vi "Format Fast Data Files.vi"() -> ()   [LabVIEW 2013]
uses:
  <vilib>/Utility/file.llb/Read From Spreadsheet File (string).vi
panel:
  out "Correct":bool
  out "Calculated Freq (Hz)":i32
  in  "stop":bool
  in  "FileName":path caption="Fast Data File to Convert Time"
  out "~Percent Formatted":dbl
  out "Processing File":bool
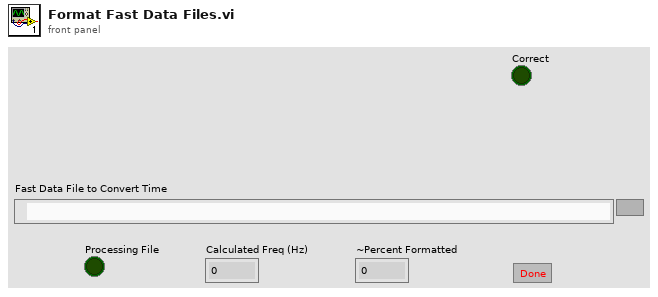
[diagram p1: front panel]
types:
  T1 = cluster{"Application":refnum<k7>, "Workbooks":refnum<k7>, "Workbook 1":refnum<k7>, "Sheets 1":refnum<k7>, "Worksheet 1":refnum<k7>, "Workbook 2":refnum<k7>, "Sheets 2":refnum<k7>, "Worksheet 2":refnum<k7>}
  T2 = cluster{"OrigFile":path, "NewFile":string, "AveFile":string, "RowIndex":i32, "Data":dbl[][], "Row#s/100":dbl, "Ave.ingLength":i32, "ExcelReferences":cluster{"Application":refnum<k7>, "Workbooks":refnum<k7>, "Workbook 1":refnum<k7>, "Sheets 1":refnum<k7>, "Worksheet 1":refnum<k7>, "Workbook 2":refnum<k7>, "Sheets 2":refnum<k7>, "Worksheet 2":refnum<k7>}, "Cells Hz":refnum<k7>, "Cells Ave":refnum<k7>, "Ave.ingPts":i32}
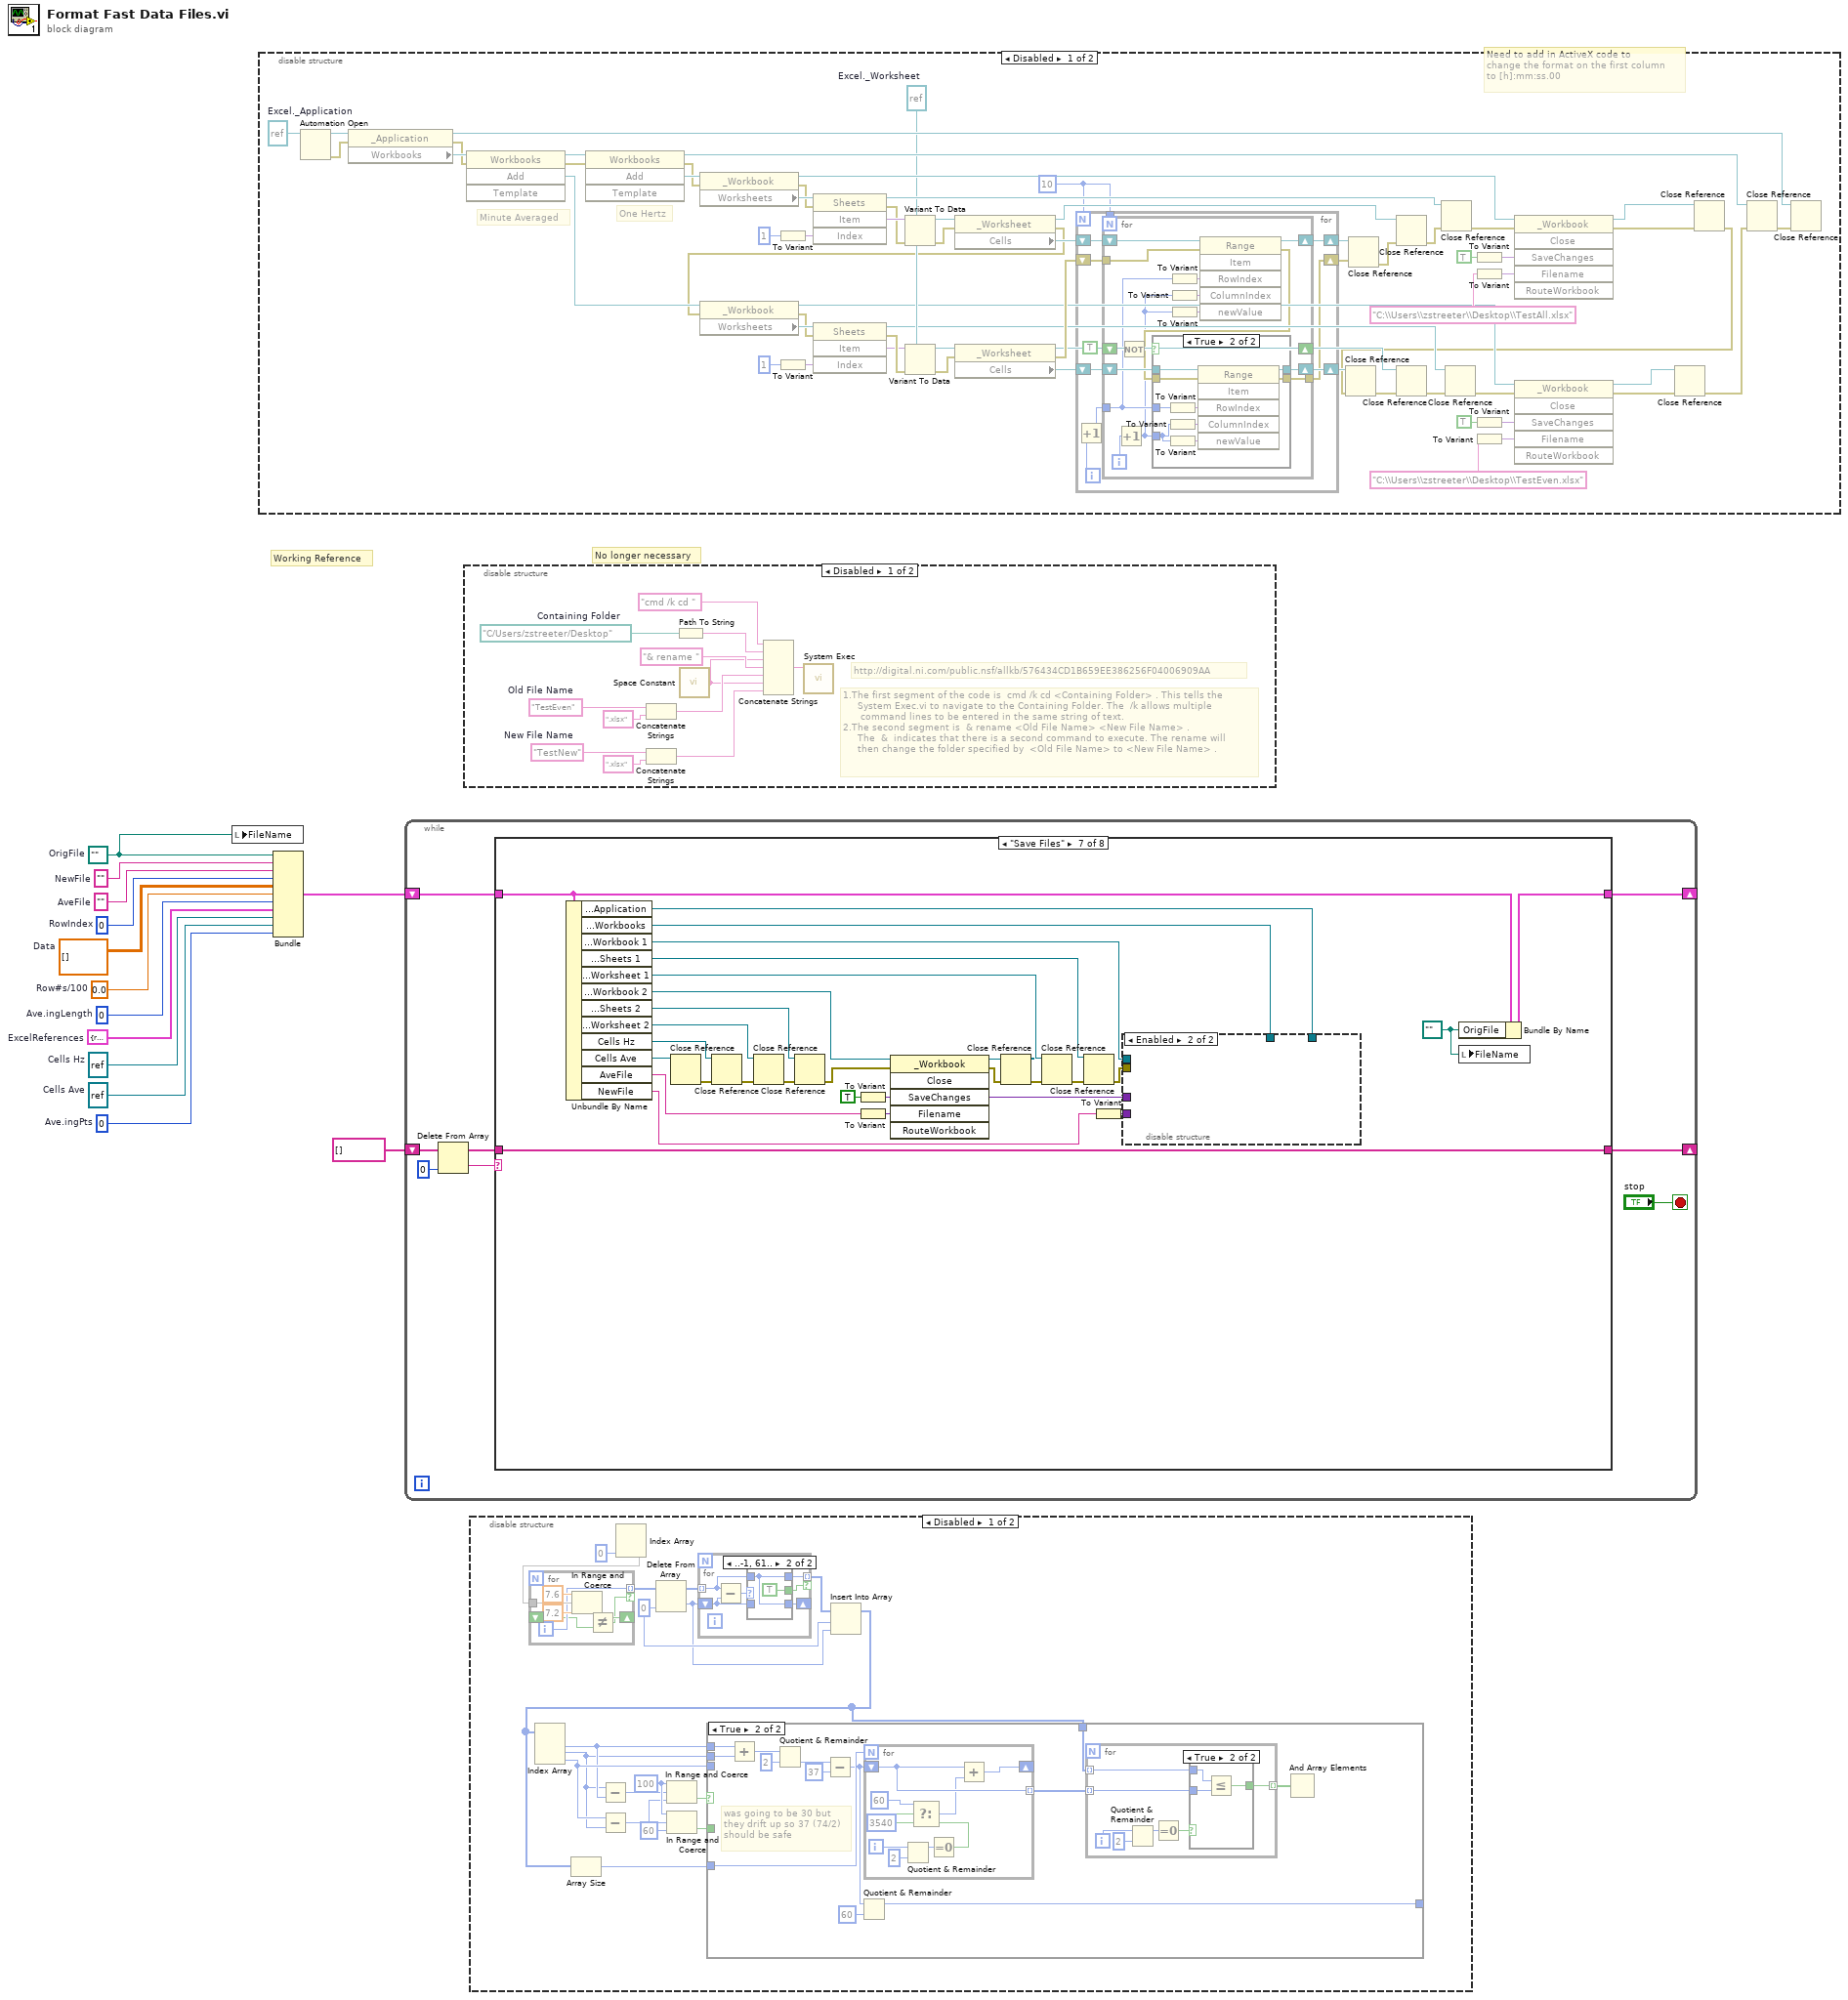
[diagram p0: block diagram]
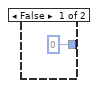
[diagram p2: hidden frame]
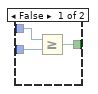
[diagram p3: hidden frame]
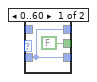
[diagram p4: hidden frame]
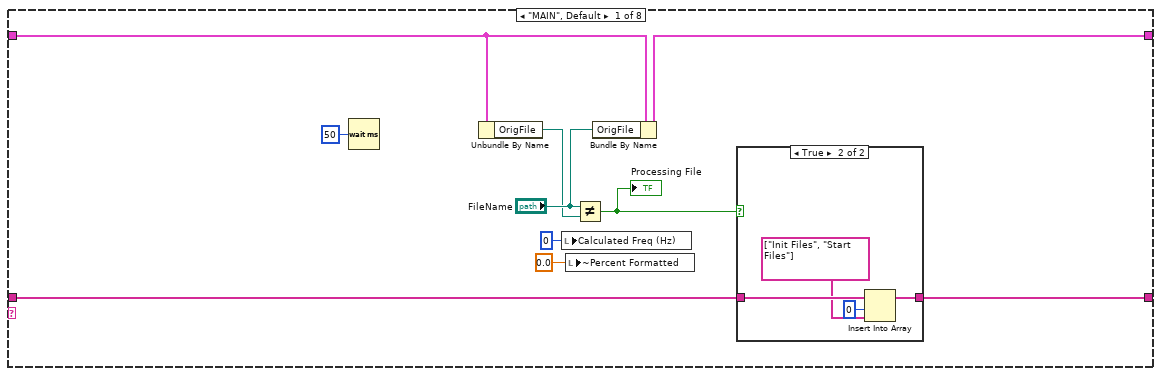
[diagram p6: hidden frame]
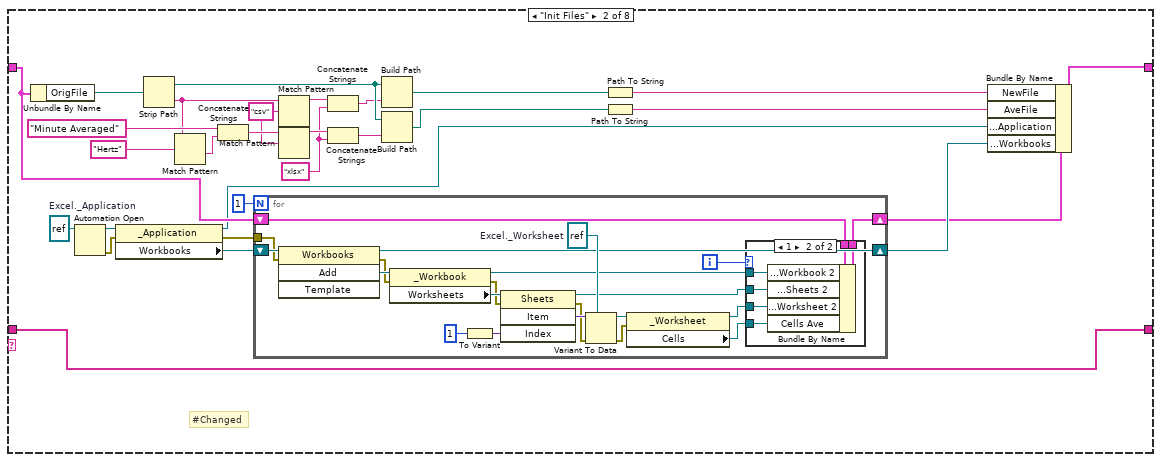
[diagram p8: hidden frame]
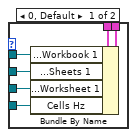
[diagram p9: hidden frame]
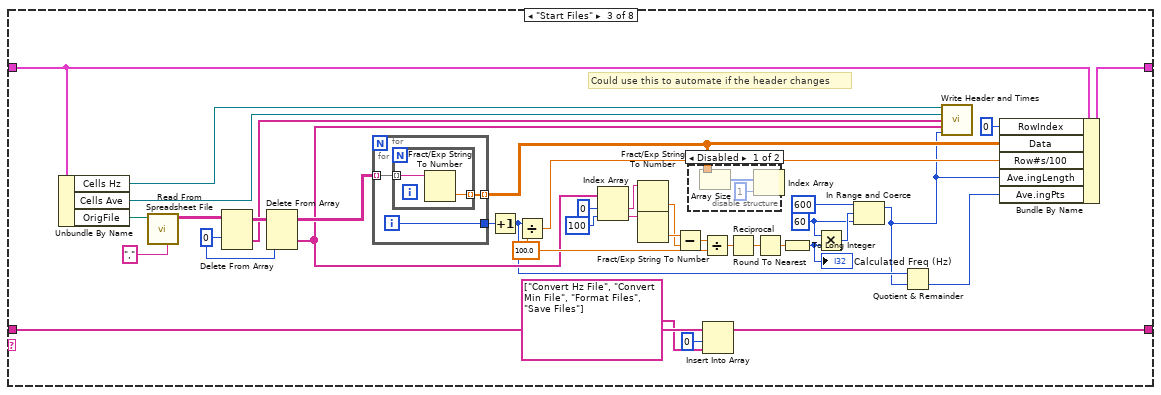
[diagram p10: hidden frame]
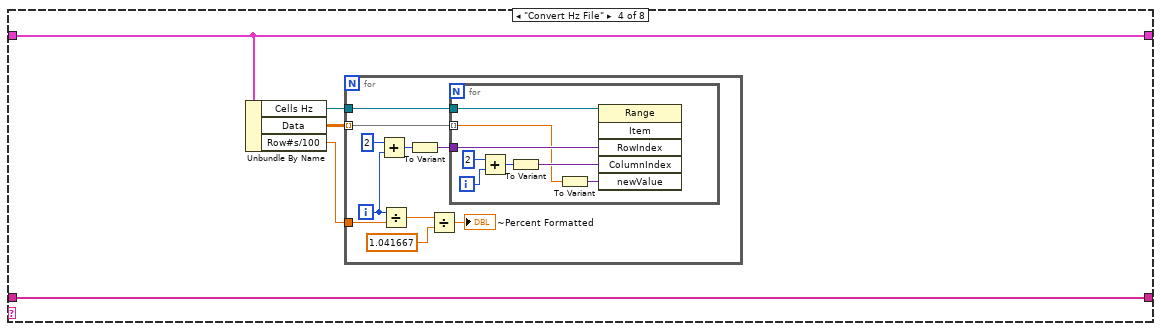
[diagram p12: hidden frame]
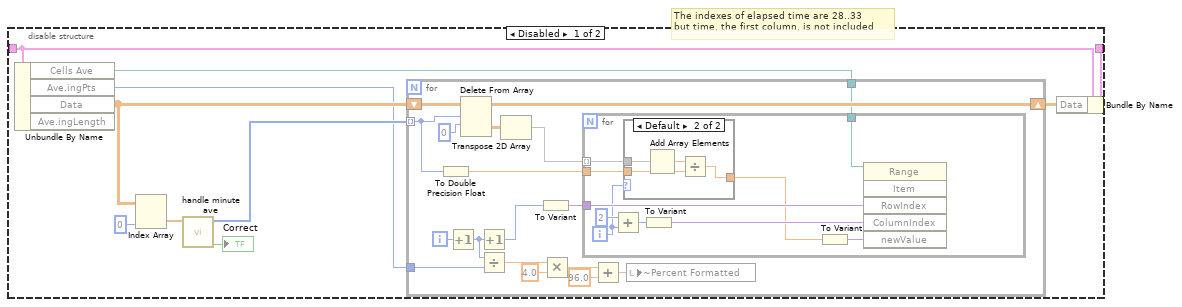
[diagram p14: hidden frame]
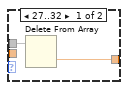
[diagram p15: hidden frame]
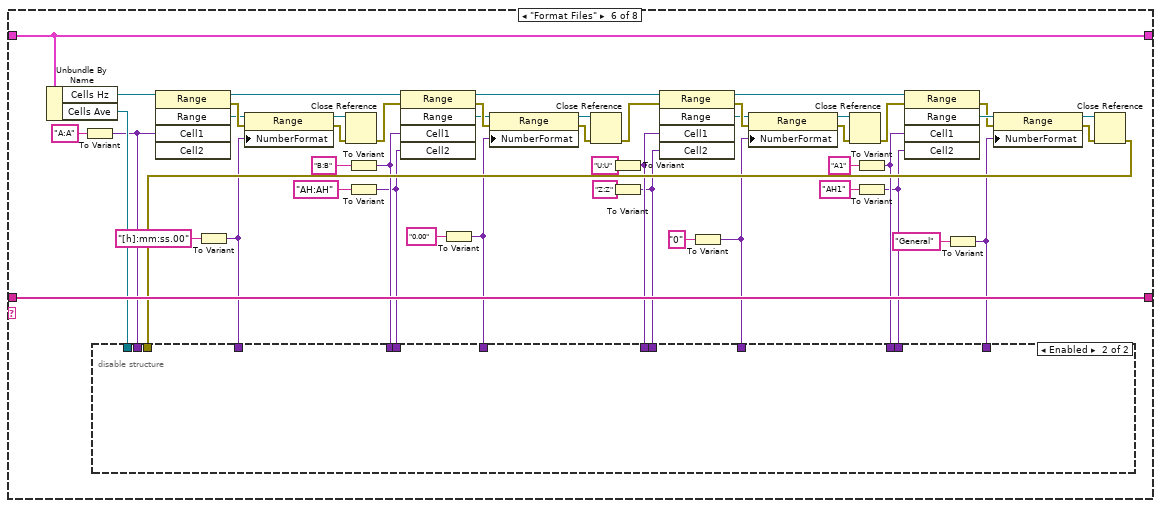
[diagram p16: hidden frame]
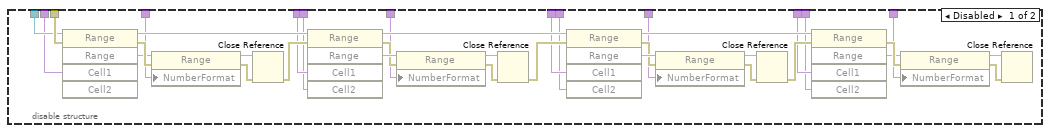
[diagram p17: hidden frame]
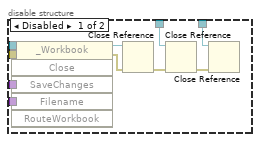
[diagram p18: hidden frame]
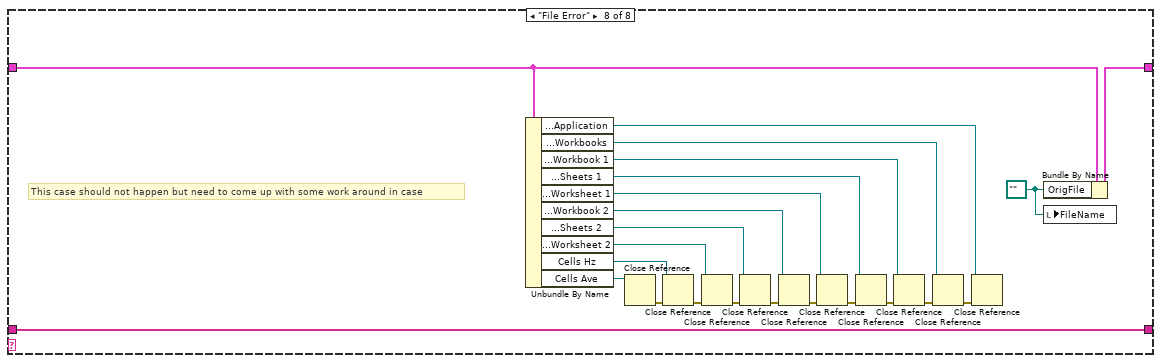
[diagram p19: hidden frame]
diagram:
  w3 = 0  # Ave.ingPts
  w5 = ""  # AveFile
  w4 = ""  # NewFile
  w6 = refnum<k7> refnum  # Cells Ave
  w7 = refnum<k7> refnum  # Cells Hz
  w8 = T1 {"Application"=refnum, "Workbooks"=refnum, "Workbook 1"=refnum, "Sheets 1"=refnum, "Worksheet 1"=refnum, "Workbook 2"=refnum, "Sheets 2"=refnum, "Worksheet 2"=refnum}  # ExcelReferences
  w10 = 0  # Ave.ingLength
  w9 = dbl[][] []  # Data
  w12 = 0  # RowIndex
  w11 = 0.0  # Row#s/100
  w2 = path ""  # OrigFile
  # "Working Reference"
  # "No longer necessary"
  n1 = local write "FileName"(w2) -> ()
  n2 = disable-structure shown="Disabled" {
    frame Disabled {
      w29 = 10
      w38 = refnum<k7> refnum  # Excel._Worksheet
      w77 = refnum<k7> refnum  # Excel._Application
      # "Need to add in ActiveX code to\nchange the format on the first column\nto [h]:mm:ss.00"
      # "Minute Averaged"
      # "One Hertz"
      n3 = Automation Open(Automation Refnum=w77) -> (Automation Refnum=w75:refnum<k7>, error out=w71:errorcluster)  [unwired: 3 in]
      n4 = property class="_Application"(reference=w75, error in=w71) -> (reference out=w64:refnum<k7>, error out=w48:errorcluster, "Workbooks"=w49:refnum<k7>)
      n5 = invoke class="Workbooks" method="Add"(reference=w49, error in=w48) -> (reference out=w46:refnum<k7>, error out=w47:errorcluster, "Add"=w45:refnum<k7>)  [unwired: 2 in, 1 out]
      n6 = invoke class="Workbooks" method="Add"(reference=w46, error in=w47) -> (reference out=w66:refnum<k7>, error out=w70:errorcluster, "Add"=w74:refnum<k7>)  [unwired: 2 in, 1 out]
      n7 = property class="_Workbook"(reference=w74, error in=w70) -> (reference out=w56:refnum<k7>, error out=w62:errorcluster, "Worksheets"=w63:refnum<k7>)
      n8 = To Variant(anything=1) -> (Variant=w59:variant)
      n9 = To Variant(anything=1) -> (Variant=w44:variant)
      n10 = invoke class="Sheets" method="Item"(reference=w63, error in=w62, "Index"=w59) -> (reference out=w67:refnum<k7>, error out=w69:errorcluster, "Item"=w72:variant)  [unwired: 1 in, 1 out]
      n11 = Variant To Data(error in=w69, type=w38, Variant=w72) -> (data=w61:refnum<k7>, error out=w68:errorcluster)
      n12 = property class="_Worksheet"(reference=w61, error in=w68) -> (reference out=w34:refnum<k7>, error out=w37:errorcluster, "Cells"=w60:refnum<k7>)
      n13 = property class="_Workbook"(reference=w45, error in=w37) -> (reference out=w19:refnum<k7>, error out=w41:errorcluster, "Worksheets"=w42:refnum<k7>)
      n14 = invoke class="Sheets" method="Item"(reference=w42, error in=w41, "Index"=w44) -> (reference out=w24:refnum<k7>, error out=w40:errorcluster, "Item"=w39:variant)  [unwired: 1 in, 1 out]
      n15 = Variant To Data(error in=w40, type=w38, Variant=w39) -> (data=w36:refnum<k7>, error out=w35:errorcluster)
      n16 = property class="_Worksheet"(reference=w36, error in=w35) -> (reference out=w25:refnum<k7>, error out=w31:errorcluster, "Cells"=w32:refnum<k7>)
      n17 = for {
        N: w29 -> [_]
        shift-right: [w86] -> w33
        shift-left: w60 -> [w87]
        shift-right: [w84] -> w28
        shift-left: w32 -> [w85]
        shift-right: [w81] -> w30
        shift-left: w31 -> [w82]
        tunnel: w29 -> [w78]
        i -> [w80]
        n18 = Increment(x=w80) -> (x+1=w79:i32)
        n19 = for {
          N: w78 -> [_]
          shift-right: [w98] -> w86
          shift-left: w87 -> [w102]
          shift-right: [w94] -> w84
          shift-left: w85 -> [w95]
          shift-right: [w96] -> _
          shift-left: TRUE -> [w97]
          tunnel: w82 -> [w93]
          tunnel: [w91] -> w81
          tunnel: w79 -> [w90]
          i -> [w89]
          n20 = Increment(x=w89) -> (x+1=w88:i32)
          n21 = Not(x=w97) -> (.not. x?=w96:bool)
          n22 = To Variant(anything=w90) -> (Variant=w99:variant)
          n23 = To Variant(anything=w88) -> (Variant=w100:variant)
          n24 = To Variant(anything=w88) -> (Variant=w101:variant)
          n25 = invoke class="Range" method="Item"(reference=w102, error in=w93, "RowIndex"=w99, "ColumnIndex"=w100, "newValue"=w101) -> (reference out=w98:refnum<k7>, error out=w92:errorcluster)  [unwired: 1 in, 4 out]
          n26 = case shown="True" w96 {
            tunnel: w95 -> [w104 w110]
            tunnel: [w104 w109] -> w94
            tunnel: w92 -> [w103 w108]
            tunnel: [w103 w107] -> w91
            tunnel: w90 -> [_ w106]
            tunnel: w88 -> [_ w105]
            frame False {
            }
            frame True {
              n27 = To Variant(anything=w106) -> (Variant=w113:variant)
              n28 = To Variant(anything=w105) -> (Variant=w112:variant)
              n29 = To Variant(anything=w105) -> (Variant=w111:variant)
              n30 = invoke class="Range" method="Item"(reference=w110, error in=w108, "RowIndex"=w113, "ColumnIndex"=w112, "newValue"=w111) -> (reference out=w109:refnum<k7>, error out=w107:errorcluster)  [unwired: 1 in, 4 out]
            }
          }
        }
      }
      n31 = Close Reference(reference=w33, error in (no error)=w30) -> (error out=w58:errorcluster)
      n32 = Close Reference(reference=w34, error in (no error)=w58) -> (error out=w76:errorcluster)
      n33 = Close Reference(reference=w67, error in (no error)=w76) -> (error out=w55:errorcluster)
      n34 = To Variant(anything=TRUE) -> (Variant=w51:variant)
      n35 = To Variant(anything="C:\\Users\\zstreeter\\Desktop\\TestAll.xlsx") -> (Variant=w52:variant)
      n36 = To Variant(anything=TRUE) -> (Variant=w22:variant)
      n37 = To Variant(anything="C:\\Users\\zstreeter\\Desktop\\TestEven.xlsx") -> (Variant=w21:variant)
      n38 = invoke class="_Workbook" method="Close"(reference=w56, error in=w55, "SaveChanges"=w51, "Filename"=w52) -> (reference out=w54:refnum<k7>, error out=w53:errorcluster)  [unwired: 2 in, 4 out]
      n39 = Close Reference(reference=w54, error in (no error)=w53) -> (error out=w15:errorcluster)
      n40 = Close Reference(reference=w28, error in (no error)=w15) -> (error out=w27:errorcluster)
      n41 = Close Reference(reference=w25, error in (no error)=w27) -> (error out=w26:errorcluster)
      n42 = Close Reference(reference=w24, error in (no error)=w26) -> (error out=w18:errorcluster)
      n43 = invoke class="_Workbook" method="Close"(reference=w19, error in=w18, "SaveChanges"=w22, "Filename"=w21) -> (reference out=w17:refnum<k7>, error out=w16:errorcluster)  [unwired: 2 in, 4 out]
      n44 = Close Reference(reference=w17, error in (no error)=w16) -> (error out=w14:errorcluster)
      n45 = Close Reference(reference=w66, error in (no error)=w14) -> (error out=w65:errorcluster)
      n46 = Close Reference(reference=w64, error in (no error)=w65) -> ()  [unwired: 1 out]
    }
    frame Enabled {
    }
  }
  n47 = Bundle("OrigFile"=w2, "NewFile"=w4, "AveFile"=w5, "RowIndex"=w12, "Data"=w9, "Row#s/100"=w11, "Ave.ingLength"=w10, "ExcelReferences"=w8, "Cells Hz"=w7, "Cells Ave"=w6, "Ave.ingPts"=w3) -> (w13:T2)  [unwired: 1 in]
  n48 = while {
    shift-right: [w117] -> _
    shift-left: string[] [] -> [w121]
    shift-right: [w115] -> _
    shift-left: w13 -> [w116]
    stop <- "stop" stop-if-true
    n49 = Delete From Array(array=w121, index=0) -> (deleted portion=w119:string, array with subset deleted=w118:string[])  [unwired: 1 in]
    n50 = case shown="\"Save Files\"" w119 {
      tunnel: w118 -> [w126 w164 w236 w249 w270 w364 w428 w461]
      tunnel: [w125 w164 w235 w249 w270 w364 w428 w461] -> w117
      tunnel: w116 -> [w130 w163 w234 w248 w269 w363 w427 w440]
      tunnel: [w129 w165 w233 w248 w268 w363 w426 w439] -> w115
      frame "MAIN", Default {
        n51 = Wait (ms)(milliseconds to wait=u32 50) -> ()  [unwired: 1 out]
        n52 = Unbundle By Name(w130) -> ("OrigFile"=w127:path)
        n53 = local write "Calculated Freq (Hz)"(0 ("Calculated Freq (Hz)")) -> ()
        n54 = local write "~Percent Formatted"(0.0 ("~Percent Formatted 2")) -> ()
        n55 = Not Equal?(x="FileName", y=w127) -> (x != y?=w124:bool)
        "Processing File" <- w124
        n56 = Bundle By Name(cluster=w130, "OrigFile"="FileName") -> (w129:T2)
        n57 = case shown="True" w124 {
          tunnel: w126 -> [w132 w136]
          tunnel: [w132 w135] -> w125
          frame False {
          }
          frame True {
            n58 = Insert Into Array(array=w136, index=0, new element=string[] ["Init Files", "Start Files"]) -> (w135:string[])
          }
        }
      }
      frame "Init Files" {
        w141 = refnum<k7> refnum  # Excel._Application
        w152 = "xlsx" ("regular expression")
        w156 = "csv" ("regular expression")
        # "#Changed"
        n59 = Unbundle By Name(w163) -> ("OrigFile"=w158:path)
        n60 = Automation Open(Automation Refnum=w141) -> (Automation Refnum=w142:refnum<k7>, error out=w143:errorcluster)  [unwired: 3 in]
        n61 = property class="_Application"(reference=w142, error in=w143) -> (reference out=w139:refnum<k7>, error out=w145:errorcluster, "Workbooks"=w144:refnum<k7>)
        n62 = Strip Path(path=w158) -> (stripped path=w162:path, name=w155:string)
        n63 = Match Pattern(string=w155, regular expression="Hertz") -> (after substring=w160:string)  [unwired: 1 in, 3 out]
        n64 = Concatenate Strings("Minute Averaged" ("string"), w160) -> (w157:string)
        n65 = for {
          N: 1 -> [_]
          shift-right: [w173] -> w140
          shift-left: w144 -> [w176]
          tunnel: w145 -> [w175]
          shift-right: [w171] -> w138
          shift-left: w163 -> [w172]
          i -> [w166]
          w174 = refnum<k7> refnum  # Excel._Worksheet
          n66 = invoke class="Workbooks" method="Add"(reference=w176, error in=w175) -> (reference out=w173:refnum<k7>, error out=w183:errorcluster, "Add"=w186:refnum<k7>)  [unwired: 2 in, 1 out]
          n67 = property class="_Workbook"(reference=w186, error in=w183) -> (reference out=w170:refnum<k7>, error out=w179:errorcluster, "Worksheets"=w180:refnum<k7>)
          n68 = To Variant(anything=1) -> (Variant=w177:variant)
          n69 = invoke class="Sheets" method="Item"(reference=w180, error in=w179, "Index"=w177) -> (reference out=w169:refnum<k7>, error out=w182:errorcluster, "Item"=w184:variant)  [unwired: 1 in, 1 out]
          n70 = Variant To Data(error in=w182, type=w174, Variant=w184) -> (data=w178:refnum<k7>, error out=w181:errorcluster)
          n71 = property class="_Worksheet"(reference=w178, error in=w181) -> (reference out=w168:refnum<k7>, "Cells"=w167:refnum<k7>)  [unwired: 1 out]
          n72 = case shown="1" w166 {
            tunnel: w172 -> [w192 w198]
            tunnel: [w191 w197] -> w171
            tunnel: w170 -> [w190 w196]
            tunnel: w169 -> [w189 w195]
            tunnel: w168 -> [w188 w194]
            tunnel: w167 -> [w187 w193]
            frame 0, Default {
              n73 = Bundle By Name(cluster=w192, "ExcelReferences.Workbook 1"=w190, "ExcelReferences.Sheets 1"=w189, "ExcelReferences.Worksheet 1"=w188, "Cells Hz"=w187) -> (w191:T2)
            }
            frame 1 {
              n74 = Bundle By Name(cluster=w198, "ExcelReferences.Workbook 2"=w196, "ExcelReferences.Sheets 2"=w195, "ExcelReferences.Worksheet 2"=w194, "Cells Ave"=w193) -> (w197:T2)
            }
          }
        }
        n75 = Match Pattern(string=w155, regular expression=w156) -> (before substring=w153:string)  [unwired: 1 in, 3 out]
        n76 = Match Pattern(string=w157, regular expression=w156) -> (before substring=w154:string)  [unwired: 1 in, 3 out]
        n77 = Concatenate Strings(w153, w152) -> (w150:string)
        n78 = Concatenate Strings(w154, w152) -> (w151:string)
        n79 = Build Path(base path=w162, name or relative path=w150) -> (appended path=w148:path)
        n80 = Build Path(base path=w162, name or relative path=w151) -> (appended path=w149:path)
        n81 = Path To String(path=w148) -> (string=w146:string)
        n82 = Path To String(path=w149) -> (string=w147:string)
        n83 = Bundle By Name(cluster=w138, "NewFile"=w146, "AveFile"=w147, "ExcelReferences.Application"=w139, "ExcelReferences.Workbooks"=w140) -> (w165:T2)
      }
      frame "Start Files" {
        w209 = 60 ("x")
        w204 = 100.0 ("y")
        w221 = 0 ("index (row)")
        # "Could use this to automate if the header changes"
        n84 = Unbundle By Name(w234) -> ("Cells Hz"=w228:refnum<k7>, "Cells Ave"=w229:refnum<k7>, "OrigFile"=w230:path)
        n85 = call-poly <vilib>:"Read From Spreadsheet File.vi"("delimiter (\\t)"="," ("delimiter (\\t)"), "file path (dialog if empty)"=w230) -> ("all rows"=w231:string[][])  [unwired: 5 in, 4 out]
        n86 = Delete From Array(array=w231, index (row)=w221) -> (deleted portion=w202:string[], array with subset deleted=w226:string[][])  [unwired: 2 in]
        n87 = Delete From Array(array=w226, index (col)=w221) -> (deleted portion=w203:string[], array with subset deleted=w222:string[][])  [unwired: 2 in]
        n88 = for {
          tunnel: w222 -> [w242] mode=indexing
          tunnel: [w241] -> w207 mode=indexing
          tunnel: [w240] -> w225
          i -> [w240]
          n89 = for {
            tunnel: w242 -> [w244] mode=indexing
            tunnel: [w243] -> w241 mode=indexing
            n90 = Fract/Exp String To Number(string=w244) -> (number=w243:dbl)  [unwired: 3 in, 1 out]
          }
        }
        n91 = Increment(x=w225) -> (x+1=w201:i32)
        n92 = Divide(x=w201, y=w204) -> (x/y=w205:dbl)
        n93 = Index Array(array=w203, index #1=0 ("index"), index #2=100 ("index")) -> (element #1=w218:string, element #2=w217:string)
        n94 = Fract/Exp String To Number(string=w218) -> (number=w215:dbl)  [unwired: 3 in, 1 out]
        n95 = Fract/Exp String To Number(string=w217) -> (number=w216:dbl)  [unwired: 3 in, 1 out]
        n96 = Subtract(x=w216, y=w215) -> (x-y=w214:dbl)
        n97 = disable-structure shown="Disabled" {
          disable-tunnel: w207 -> [w237 _]
          frame Disabled {
            n98 = Array Size(array=w237) -> (size(s)=w239:i32[])
            n99 = Index Array(array=w239, index=1) -> ()  [unwired: 1 out]
          }
          frame Enabled {
          }
        }
        n100 = Divide(x=w214, y=w204) -> (x/y=w213:dbl)
        n101 = Insert Into Array(array=w236, index=0, new element=string[] ["Convert Hz File", "Convert Min File", "Format Files", "Save Files"]) -> (w235:string[])
        n102 = Reciprocal(x=w213) -> (1/x=w212:dbl)
        n103 = Round To Nearest(number=w212) -> (nearest integer value=w211:dbl)
        n104 = To Long Integer(number=w211) -> (32bit integer=w206:i32)
        "Calculated Freq (Hz)" <- w206
        n105 = Multiply(x=w209, y=w206) -> (x*y=w210:i32)
        n106 = In Range and Coerce(upper limit=600, x=w210, lower limit=w209) -> (coerced(x)=w199:i32)  [unwired: 1 out]
        n107 = Quotient & Remainder(x=w201, y=w199) -> (floor(x/y)=w200:i32)  [unwired: 1 out]
        n108 = call "Write Header and Times.vi"("Cells Hz IN"=w228, "Cells Ave IN"=w229, "Header Array"=w202, "Time Array"=w203, "Ave.ingLength"=w199) -> ()  [unwired: 9 in, 2 out]
        n109 = Bundle By Name(cluster=w234, "RowIndex"=0, "Data"=w207, "Row#s/100"=w205, "Ave.ingLength"=w199, "Ave.ingPts"=w200) -> (w233:T2)
      }
      frame "Convert Hz File" {
        n110 = Unbundle By Name(w248) -> ("Cells Hz"=w245:refnum<k7>, "Data"=w247:dbl[][], "Row#s/100"=w246:dbl)
        n111 = for {
          tunnel: w247 -> [w259] mode=indexing
          tunnel: w246 -> [w255]
          tunnel: w245 -> [w252]
          i -> [w254]
          n112 = Add(x=2, y=w254) -> (x+y=w251:i32)
          n113 = Divide(x=w254, y=w255) -> (x/y=w256:dbl)
          n114 = To Variant(anything=w251) -> (Variant=w250:variant)
          n115 = Divide(x=w256, y=1.041667) -> (x/y=→"~Percent Formatted":dbl)
          n116 = for {
            tunnel: w259 -> [w260] mode=indexing
            tunnel: w252 -> [w267]
            tunnel: w250 -> [w266]
            i -> [w262]
            n117 = Add(x=2, y=w262) -> (x+y=w265:i32)
            n118 = To Variant(anything=w265) -> (Variant=w263:variant)
            n119 = To Variant(anything=w260) -> (Variant=w261:variant)
            n120 = invoke class="Range" method="Item"(reference=w267, "RowIndex"=w266, "ColumnIndex"=w263, "newValue"=w261) -> ()  [unwired: 2 in, 6 out]
          }
        }
      }
      frame "Convert Min File" {
        n121 = disable-structure shown="Enabled" {
          disable-tunnel: w269 -> [w280 w315]
          disable-tunnel: [w279 w315] -> w268
          frame Disabled {
            # "The indexes of elapsed time are 28..33\nbut time, the first column, is not included"
            n122 = Unbundle By Name(w280) -> ("Cells Ave"=w278:refnum<k7>, "Ave.ingPts"=w271:i32, "Data"=w275:dbl[][])  [unwired: 1 out]
            n123 = Index Array(array=w275, index (col)=0 ("disabled index (col)")) -> (element=w274:dbl[])  [unwired: 1 in]
            n124 = call "handle minute ave.vi"("Array"=w274) -> ("Correct"=→"Correct":bool, "Array 2"=w272:i32[])  [unwired: 9 in]
            n125 = for {
              shift-right: [w296] -> w277
              shift-left: w275 -> [w298]
              tunnel: w272 -> [w283] mode=indexing
              tunnel: w278 -> [w286]
              tunnel: w271 -> [w281]
              i -> [w295]
              n126 = To Double Precision Float(number=w283) -> (double precision float=w282:dbl)
              n127 = Increment(x=w295) -> (x+1=w294:i32)
              n128 = Delete From Array(array=w298, length=w283, index (row)=0) -> (deleted portion=w284:dbl[][], array with subset deleted=w296:dbl[][])  [unwired: 1 in]
              n129 = Increment(x=w294) -> (x+1=w289:i32)
              n130 = Divide(x=w294, y=w281) -> (x/y=w293:dbl)
              n131 = Transpose 2D Array(2D array=w284) -> (transposed array=w285:dbl[][])
              n132 = To Variant(anything=w289) -> (Variant=w290:variant)
              n133 = Multiply(x=w293, y=4.0) -> (x*y=w288:dbl)
              n134 = for {
                tunnel: w290 -> [w308]
                tunnel: w286 -> [w304]
                tunnel: w285 -> [w303] mode=indexing
                tunnel: w282 -> [w302]
                i -> [w301]
                n135 = Add(x=2, y=w301) -> (x+y=w307:i32)
                n136 = case shown="Default" w301 {
                  tunnel: w303 -> [w310 w313]
                  tunnel: w302 -> [_ w312]
                  tunnel: [w309 w311] -> w300
                  frame 27..32 {
                    n137 = Delete From Array(array=w310) -> (deleted portion=w309:dbl)  [unwired: 2 in, 1 out]
                  }
                  frame Default {
                    n138 = Add Array Elements(numeric array=w313) -> (sum=w314:dbl)
                    n139 = Divide(x=w314, y=w312) -> (x/y=w311:dbl)
                  }
                }
                n140 = To Variant(anything=w307) -> (Variant=w305:variant)
                n141 = To Variant(anything=w300) -> (Variant=w299:variant)
                n142 = invoke class="Range" method="Item"(reference=w304, "RowIndex"=w308, "ColumnIndex"=w305, "newValue"=w299) -> ()  [unwired: 2 in, 6 out]
              }
              n143 = Add(x=w288, y=96.0 ("x")) -> (x+y=w291:dbl)
              n144 = local write "~Percent Formatted"(w291) -> ()
            }
            n145 = Bundle By Name(cluster=w280, "Data"=w277) -> (w279:T2)
          }
          frame Enabled {
          }
        }
      }
      frame "Format Files" {
        n146 = Unbundle By Name(w363) -> ("Cells Hz"=w318:refnum<k7>, "Cells Ave"=w343:refnum<k7>)
        n147 = To Variant(anything="A:A") -> (Variant=w339:variant)
        n148 = invoke class="Range" method="Range"(reference=w318, "Cell1"=w339) -> (reference out=w317:refnum<k7>, error out=w362:errorcluster, "Range"=w316:refnum<k7>)  [unwired: 3 in, 2 out]
        n149 = To Variant(anything="[h]:mm:ss.00") -> (Variant=w325:variant)
        n150 = property class="Range"(reference=w316, error in=w362, "NumberFormat"=w325) -> (reference out=w360:refnum<k7>, error out=w361:errorcluster)
        n151 = Close Reference(reference=w360, error in (no error)=w361) -> (error out=w347:errorcluster)
        n152 = To Variant(anything="B:B") -> (Variant=w336:variant)
        n153 = To Variant(anything="AH:AH") -> (Variant=w335:variant)
        n154 = invoke class="Range" method="Range"(reference=w317, error in=w347, "Cell1"=w336, "Cell2"=w335) -> (reference out=w342:refnum<k7>, error out=w357:errorcluster, "Range"=w356:refnum<k7>)  [unwired: 1 in, 2 out]
        n155 = To Variant(anything="0.00") -> (Variant=w319:variant)
        n156 = property class="Range"(reference=w356, error in=w357, "NumberFormat"=w319) -> (reference out=w359:refnum<k7>, error out=w358:errorcluster)
        n157 = Close Reference(reference=w359, error in (no error)=w358) -> (error out=w346:errorcluster)
        n158 = To Variant(anything="U:U") -> (Variant=w328:variant)
        n159 = To Variant(anything="Z:Z") -> (Variant=w327:variant)
        n160 = invoke class="Range" method="Range"(reference=w342, error in=w346, "Cell1"=w328, "Cell2"=w327) -> (reference out=w341:refnum<k7>, error out=w349:errorcluster, "Range"=w348:refnum<k7>)  [unwired: 1 in, 2 out]
        n161 = To Variant(anything="0") -> (Variant=w320:variant)
        n162 = property class="Range"(reference=w348, error in=w349, "NumberFormat"=w320) -> (reference out=w351:refnum<k7>, error out=w350:errorcluster)
        n163 = Close Reference(reference=w351, error in (no error)=w350) -> (error out=w345:errorcluster)
        n164 = To Variant(anything="A1") -> (Variant=w330:variant)
        n165 = To Variant(anything="AH1") -> (Variant=w329:variant)
        n166 = invoke class="Range" method="Range"(reference=w341, error in=w345, "Cell1"=w330, "Cell2"=w329) -> (error out=w354:errorcluster, "Range"=w355:refnum<k7>)  [unwired: 1 in, 3 out]
        n167 = To Variant(anything="General") -> (Variant=w323:variant)
        n168 = property class="Range"(reference=w355, error in=w354, "NumberFormat"=w323) -> (reference out=w352:refnum<k7>, error out=w353:errorcluster)
        n169 = Close Reference(reference=w352, error in (no error)=w353) -> (error out=w344:errorcluster)
        n170 = disable-structure shown="Enabled" {
          disable-tunnel: w344 -> [w383 _]
          disable-tunnel: w343 -> [w379 _]
          disable-tunnel: w339 -> [w375 _]
          disable-tunnel: w336 -> [w374 _]
          disable-tunnel: w335 -> [w373 _]
          disable-tunnel: w330 -> [w372 _]
          disable-tunnel: w329 -> [w371 _]
          disable-tunnel: w328 -> [w370 _]
          disable-tunnel: w327 -> [w369 _]
          disable-tunnel: w325 -> [w368 _]
          disable-tunnel: w323 -> [w367 _]
          disable-tunnel: w320 -> [w366 _]
          disable-tunnel: w319 -> [w365 _]
          frame Disabled {
            n171 = invoke class="Range" method="Range"(reference=w379, error in=w383, "Cell1"=w375) -> (reference out=w378:refnum<k7>, error out=w385:errorcluster, "Range"=w384:refnum<k7>)  [unwired: 2 in, 2 out]
            n172 = property class="Range"(reference=w384, error in=w385, "NumberFormat"=w368) -> (reference out=w387:refnum<k7>, error out=w386:errorcluster)
            n173 = Close Reference(reference=w387, error in (no error)=w386) -> (error out=w382:errorcluster)
            n174 = invoke class="Range" method="Range"(reference=w378, error in=w382, "Cell1"=w374, "Cell2"=w373) -> (reference out=w377:refnum<k7>, error out=w390:errorcluster, "Range"=w391:refnum<k7>)  [unwired: 1 in, 2 out]
            n175 = property class="Range"(reference=w391, error in=w390, "NumberFormat"=w365) -> (reference out=w388:refnum<k7>, error out=w389:errorcluster)
            n176 = Close Reference(reference=w388, error in (no error)=w389) -> (error out=w381:errorcluster)
            n177 = invoke class="Range" method="Range"(reference=w377, error in=w381, "Cell1"=w370, "Cell2"=w369) -> (reference out=w376:refnum<k7>, error out=w398:errorcluster, "Range"=w399:refnum<k7>)  [unwired: 1 in, 2 out]
            n178 = property class="Range"(reference=w399, error in=w398, "NumberFormat"=w366) -> (reference out=w396:refnum<k7>, error out=w397:errorcluster)
            n179 = Close Reference(reference=w396, error in (no error)=w397) -> (error out=w380:errorcluster)
            n180 = invoke class="Range" method="Range"(reference=w376, error in=w380, "Cell1"=w372, "Cell2"=w371) -> (error out=w393:errorcluster, "Range"=w392:refnum<k7>)  [unwired: 1 in, 3 out]
            n181 = property class="Range"(reference=w392, error in=w393, "NumberFormat"=w367) -> (reference out=w395:refnum<k7>, error out=w394:errorcluster)
            n182 = Close Reference(reference=w395, error in (no error)=w394) -> ()  [unwired: 1 out]
          }
          frame Enabled {
          }
        }
      }
      frame "Save Files" {
        w400 = path "" ("OrigFile")
        n183 = Unbundle By Name(w427) -> ("ExcelReferences.Application"=w418:refnum<k7>, "ExcelReferences.Workbooks"=w419:refnum<k7>, "ExcelReferences.Workbook 1"=w409:refnum<k7>, "ExcelReferences.Sheets 1"=w420:refnum<k7>, "ExcelReferences.Worksheet 1"=w421:refnum<k7>, "ExcelReferences.Workbook 2"=w408:refnum<k7>, "ExcelReferences.Sheets 2"=w422:refnum<k7>, "ExcelReferences.Worksheet 2"=w423:refnum<k7>, "Cells Hz"=w424:refnum<k7>, "Cells Ave"=w425:refnum<k7>, "AveFile"=w402:string, "NewFile"=w401:string)
        n184 = Close Reference(reference=w425) -> (error out=w417:errorcluster)  [unwired: 1 in]
        n185 = Close Reference(reference=w424, error in (no error)=w417) -> (error out=w416:errorcluster)
        n186 = Close Reference(reference=w423, error in (no error)=w416) -> (error out=w415:errorcluster)
        n187 = Close Reference(reference=w422, error in (no error)=w415) -> (error out=w406:errorcluster)
        n188 = To Variant(anything=TRUE) -> (Variant=w403:variant)
        n189 = To Variant(anything=w402) -> (Variant=w411:variant)
        n190 = invoke class="_Workbook" method="Close"(reference=w408, error in=w406, "SaveChanges"=w403, "Filename"=w411) -> (reference out=w407:refnum<k7>, error out=w405:errorcluster)  [unwired: 2 in, 4 out]
        n191 = Close Reference(reference=w407, error in (no error)=w405) -> (error out=w414:errorcluster)
        n192 = Close Reference(reference=w421, error in (no error)=w414) -> (error out=w413:errorcluster)
        n193 = Close Reference(reference=w420, error in (no error)=w413) -> (error out=w404:errorcluster)
        n194 = To Variant(anything=w401) -> (Variant=w412:variant)
        n195 = disable-structure shown="Enabled" {
          disable-tunnel: w419 -> [w438 _]
          disable-tunnel: w418 -> [w437 _]
          disable-tunnel: w412 -> [w434 _]
          disable-tunnel: w409 -> [w433 _]
          disable-tunnel: w404 -> [w431 _]
          disable-tunnel: w403 -> [w429 _]
          frame Disabled {
            n196 = invoke class="_Workbook" method="Close"(reference=w433, error in=w431, "SaveChanges"=w429, "Filename"=w434) -> (reference out=w432:refnum<k7>, error out=w430:errorcluster)  [unwired: 2 in, 4 out]
            n197 = Close Reference(reference=w432, error in (no error)=w430) -> (error out=w436:errorcluster)
            n198 = Close Reference(reference=w438, error in (no error)=w436) -> (error out=w435:errorcluster)
            n199 = Close Reference(reference=w437, error in (no error)=w435) -> ()  [unwired: 1 out]
          }
          frame Enabled {
          }
        }
        n200 = Bundle By Name(cluster=w427, "OrigFile"=w400) -> (w426:T2)
        n201 = local write "FileName"(w400) -> ()
      }
      frame "File Error" {
        w441 = path "" ("OrigFile")
        # "This case should not happen but need to come up with some work around in case"
        n202 = Unbundle By Name(w440) -> ("ExcelReferences.Application"=w451:refnum<k7>, "ExcelReferences.Workbooks"=w452:refnum<k7>, "ExcelReferences.Workbook 1"=w453:refnum<k7>, "ExcelReferences.Sheets 1"=w454:refnum<k7>, "ExcelReferences.Worksheet 1"=w455:refnum<k7>, "ExcelReferences.Workbook 2"=w456:refnum<k7>, "ExcelReferences.Sheets 2"=w457:refnum<k7>, "ExcelReferences.Worksheet 2"=w458:refnum<k7>, "Cells Hz"=w459:refnum<k7>, "Cells Ave"=w460:refnum<k7>)
        n203 = Close Reference(reference=w460) -> (error out=w450:errorcluster)  [unwired: 1 in]
        n204 = Close Reference(reference=w459, error in (no error)=w450) -> (error out=w449:errorcluster)
        n205 = Close Reference(reference=w458, error in (no error)=w449) -> (error out=w448:errorcluster)
        n206 = Close Reference(reference=w457, error in (no error)=w448) -> (error out=w447:errorcluster)
        n207 = Close Reference(reference=w456, error in (no error)=w447) -> (error out=w446:errorcluster)
        n208 = Close Reference(reference=w455, error in (no error)=w446) -> (error out=w445:errorcluster)
        n209 = Close Reference(reference=w454, error in (no error)=w445) -> (error out=w444:errorcluster)
        n210 = Close Reference(reference=w453, error in (no error)=w444) -> (error out=w443:errorcluster)
        n211 = Close Reference(reference=w452, error in (no error)=w443) -> (error out=w442:errorcluster)
        n212 = Close Reference(reference=w451, error in (no error)=w442) -> ()  [unwired: 1 out]
        n213 = Bundle By Name(cluster=w440, "OrigFile"=w441) -> (w439:T2)
        n214 = local write "FileName"(w441) -> ()
      }
    }
  }
  n215 = disable-structure shown="Disabled" {
    frame Disabled {
      w469 = "TestEven"  # Old File Name
      w471 = path "C:/Users/zstreeter/Desktop"  # Containing Folder
      w473 = "TestNew"  # New File Name
      # "http://digital.ni.com/public.nsf/allkb/576434CD1B659EE386256F04006909AA"
      # "1.The first segment of the code is  cmd /k cd <Containing Folder> . This tells the\n     System Exec.vi to navigate to the Containing Folder. The  /k allows multiple\n      command lines to be entered in the same string of text.\n2.The second segment is  & rename <Old File Name> <New File Name> . \n     The  &  indicates that there is a second command to execute. The rename will\n     then change the folder specified by  <Old File Name> to <New File Name> ."
      n216 = Concatenate Strings(w469, ".xlsx" ("string")) -> (w468:string)
      n217 = Concatenate Strings(w473, ".xlsx" ("string")) -> (w467:string)
      n218 = Path To String(path=w471) -> (string=w464:string)
      n219 = call <vilib>:"Space Constant.vi"() -> ("String"=w465:string)
      n220 = Concatenate Strings "Concatenate Strings"("cmd /k cd " ("string"), w464, w465, "& rename " ("string"), w468, w465, w467) -> (w462:string)
      n221 = call <vilib>:"System Exec.vi"("command line"=w462) -> ()  [unwired: 7 in, 4 out]
    }
    frame Enabled {
    }
  }
  n222 = disable-structure shown="Disabled" {
    frame Disabled {
      w484 = 100 ("upper limit")
      w483 = 60 ("lower limit")
      w480 = 0 ("index")
      n223 = Index Array(index (col)=0 ("disabled index (col)")) -> (element=w475)  [unwired: 2 in]
      n224 = for {
        tunnel: w475 -> [w545]
        tunnel: [w542] -> w476 mode=indexing if=w539
        shift-right: [w540] -> _
        shift-left: _ -> [w541]
        i -> [w542]
        n225 = In Range and Coerce(upper limit=7.6, x=w545, lower limit=7.2) -> (In Range?=w540:bool)  [unwired: 1 out]
        n226 = Not Equal?(x=w540, y=w541) -> (x != y?=w539:bool)
      }
      n227 = Delete From Array(array=w476, index=w480) -> (deleted portion=w479:i32, array with subset deleted=w477:i32[])  [unwired: 1 in]
      n228 = for {
        tunnel: w477 -> [w532] mode=indexing
        shift-right: [w531] -> _
        shift-left: w479 -> [w533]
        tunnel: [w530] -> w478 mode=indexing if=w529
        n229 = Subtract(x=w532, y=w533) -> (x-y=w534:i32)
        n230 = case shown="..-1, 61.." w534 {
          tunnel: w533 -> [w536 _]
          tunnel: w532 -> [_ w538]
          tunnel: [w536 w538] -> w531
          tunnel: [w536 w538] -> w530
          tunnel: [FALSE TRUE] -> w529
          frame 0..60 {
          }
          frame ..-1, 61.. {
          }
        }
      }
      n231 = Insert Into Array(array=w478, index=w480, new element=w479) -> (w491:i32[])
      n232 = Index Array(array=w491) -> (element #1=w489:i32, element #2=w488:i32, element #3=w490:i32)  [unwired: 3 in]
      n233 = Array Size(array=w491) -> (size(s)=w487:i32)
      n234 = Subtract(x=w488, y=w489) -> (x-y=w481:i32)
      n235 = Subtract(x=w490, y=w488) -> (x-y=w482:i32)
      n236 = In Range and Coerce(upper limit=w484, x=w481, lower limit=w483) -> (In Range?=w485:bool)  [unwired: 1 out]
      n237 = In Range and Coerce(upper limit=w484, x=w482, lower limit=w483) -> (In Range?=w486:bool)  [unwired: 1 out]
      n238 = case shown="True" w485 {
        tunnel: w486 -> [_ _]
        tunnel: w489 -> [_ w506]
        tunnel: w488 -> [_ w505]
        tunnel: w490 -> [_ _]
        tunnel: w487 -> [_ w500]
        tunnel: w491 -> [_ w499]
        tunnel: [0 w493] -> _
        frame False {
        }
        frame True {
          # "was going to be 30 but\nthey drift up so 37 (74/2)\nshould be safe"
          n239 = Add(x=w506, y=w505) -> (x+y=w504:i32)
          n240 = Quotient & Remainder(x=w504, y=2) -> (floor(x/y)=w502:i32)  [unwired: 1 out]
          n241 = Subtract(x=w502, y=37) -> (x-y=w495:i32)
          n242 = Quotient & Remainder(x=w495, y=60) -> (x-y*floor(x/y)=w493:i32)  [unwired: 1 out]
          n243 = for {
            N: w500 -> [_]
            shift-right: [w525] -> _
            shift-left: w495 -> [w524]
            tunnel: [w524] -> w498 mode=indexing
            i -> [w527]
            n244 = Quotient & Remainder(x=w527, y=2) -> (x-y*floor(x/y)=w526:i32)  [unwired: 1 out]
            n245 = Equal To 0?(x=w526) -> (x = 0?=w523:bool)
            n246 = Select(t=60 ("lower limit"), s=w523, f=3540) -> (s? t:f=w522:i32)
            n247 = Add(x=w524, y=w522) -> (x+y=w525:i32)
          }
          n248 = for {
            tunnel: w499 -> [w509] mode=indexing
            tunnel: w498 -> [w508] mode=indexing
            tunnel: [w507] -> w497 mode=indexing
            i -> [w511]
            n249 = Quotient & Remainder(x=w511, y=2) -> (x-y*floor(x/y)=w513:i32)  [unwired: 1 out]
            n250 = Equal To 0?(x=w513) -> (x = 0?=w510:bool)
            n251 = case shown="True" w510 {
              tunnel: w509 -> [w516 w519]
              tunnel: w508 -> [w515 w518]
              tunnel: [w514 w517] -> w507
              frame False {
                n252 = Greater Or Equal?(x=w516, y=w515) -> (x >= y?=w514:bool)
              }
              frame True {
                n253 = Less Or Equal?(x=w519, y=w518) -> (x <= y?=w517:bool)
              }
            }
          }
          n254 = And Array Elements(Boolean array=w497) -> (logical AND=w496:bool)
        }
      }
    }
    frame Enabled {
    }
  }
